vi "RefNumsDriverStation.vi"() -> ()   [LabVIEW 2018]
panel:
  out "Super_Test_Mode":bool
  out "Master_Safety_Override":bool
  out "DS Elevator Buttons":T1
  out "J1-RightY":dbl
  out "J1-View":bool
  out "J1-Left_Trigger":dbl
  out "J1-Right_Trigger":dbl
  out "J1-RightX":dbl
  out "J1-LeftY":dbl
  out "J1-DPAD":i16
  out "J1-Menu":bool
  out "J1-U":bool
  out "J1-Right_Joystick_Button":bool
  out "J1-Left_Joystick_Button":bool
  out "J1-Left_Bumper":bool
  out "J1-Right_Bumper":bool
  out "J1-Y":bool
  out "J1-X":bool
  out "J1-B":bool
  out "J1-A":bool
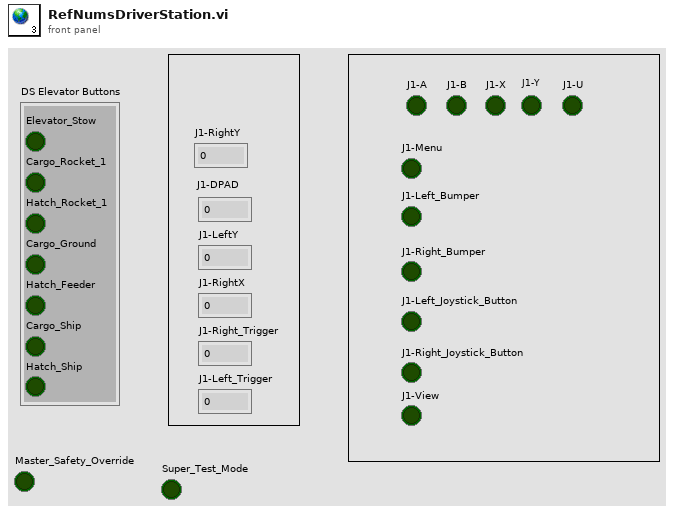
[diagram p1: front panel]
types:
  T1 = cluster{"Elevator_Stow":bool, "Cargo_Rocket_1":bool, "Hatch_Rocket_1":bool, "Cargo_Ground":bool, "Hatch_Feeder":bool, "Cargo_Ship":bool, "Hatch_Ship":bool}
diagram:
